vi "Act.vi"(8 "error in (no error)":errorcluster, 9 "VI Refnum in":refnum<vi>, 10 "Flex Msg type":refnum<class "Flex Msg.lvclass">, 11 "Get Controls in":refnum<class "Get Controls.lvclass">) -> (0 "error out":errorcluster, 1 "Await user action?":bool, 3 "Get Controls out":refnum<class "Get Controls.lvclass">)   [LabVIEW 2020, in "Msg.lvlib" / "Get Controls.lvclass"]
doc: "This implementation retrieves the control data and enqueues it on the provided queue and does not wait for user action."
uses:
  Get Controls.lvclass
  Flex Msg.lvclass
  Get Controls.lvclass/Get Controls.ctl
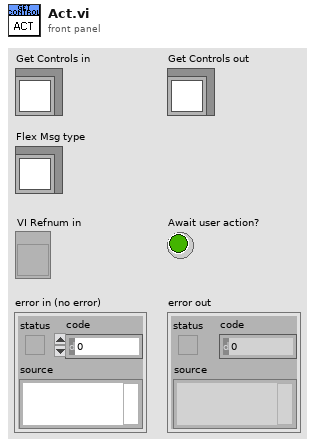
[diagram p1: front panel]
types:
  T1 = typedef "Msg.lvlib/Ctl_Control Element.ctl" = cluster{"Index":i32, "Label":string, "Value":variant}
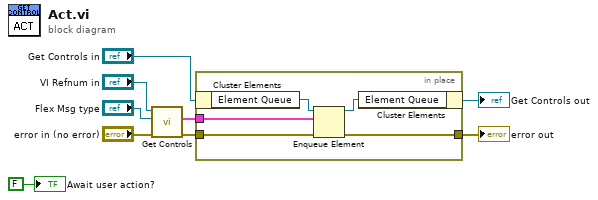
[diagram p0: block diagram]
diagram:
  n1 = call "Get Controls.vi"("error in (no error)"="error in (no error)", "Flex Msg in"="Flex Msg type", "VI Refnum in"="VI Refnum in") -> ("error out"=w2:errorcluster, "Control Element Array"=w3:T1[])  [unwired: 6 in, 1 out]
  n2 = in-place {
    in-place-border: w3 -> [w12]
    in-place-border: w2 -> [w11]
    in-place-border: [w10] -> w1
    n3 = in-place-cluster #1("Get Controls in") -> ("Element Queue"=w14:refnum<queue>)
    n4 = Enqueue Element(queue=w14, element=w12, error in (no error)=w11) -> (queue out=w13:refnum<queue>, error out=w10:errorcluster)  [unwired: 1 in, 1 out]
    n5 = in-place-cluster #1("Element Queue"=w13) -> (→"Get Controls out":refnum<class "Get Controls.lvclass">)
  }
  "error out" <- w1
  "Await user action?" <- FALSE ("Await user action?")
